vi "Read Mean.vi"(11 "VoltageResultIn":refnum<class "VoltageResult.lvclass">) -> (2 "Mean":dbl, 3 "VoltageResultOut":refnum<class "VoltageResult.lvclass">)   [LabVIEW 2020, in "VoltageResult.lvclass"]
uses:
  VoltageResult.lvclass
  VoltageResult.lvclass/VoltageResult.ctl
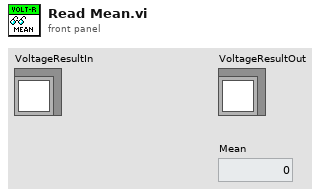
[diagram p1: front panel]
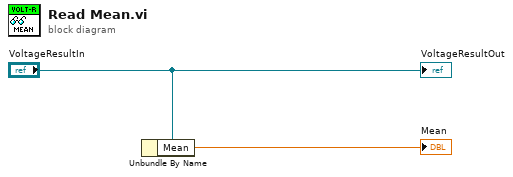
[diagram p0: block diagram]
diagram:
  n1 = Unbundle By Name("VoltageResultIn") -> ("Mean"=→"Mean":dbl)
  "VoltageResultOut" <- "VoltageResultIn"
